vi "GUI process burst data.vi"(9 "Analysis.algo":string, 10 "TXRX data":T1, 11 "WaveformGraph in":refnum<vi>) -> (2 "Result param":string[][](array[string]), 3 "Result plot":cluster{"x0":dbl, "dx":dbl, "y":dbl[]}[](array[cluster]))   [LabVIEW 2019, in "GUI.lvlib"]
uses:
  GUI.lvlib
  SubVIs/mmWave data_class/mmWave data.lvclass
  <vilib>/Analysis/4window.llb/windowTd.ctl
  <vilib>/Analysis/coordinate.llb/Angle Units.ctl
  <vilib>/Analysis/2dsp.llb/1D Convolution (CDB).vi
  <vilib>/Analysis/coordinate.llb/Wrap Angle (array).vi
  <vilib>/measure/maspectr.llb/FFT Spectrum (Mag-Phase) for 1 Chan (CDB).vi
  <vilib>/Analysis/NI_AALPro.lvlib
  <vilib>/Analysis/NI_AAL_Angle.lvlib
  <vilib>/measure/NI_MAPro.lvlib
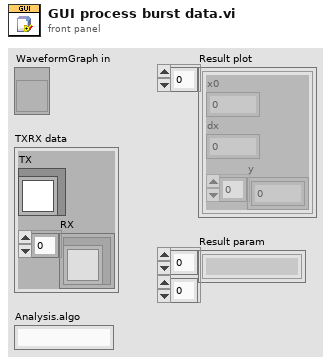
[diagram p1: front panel]
types:
  T1 = cluster{"TX":refnum<class "mmWave data.lvclass">, "RX":refnum<class "mmWave data.lvclass">[]}
  T2 = cluster{"dB On (F)":bool, "unwrap phase (F)":bool, "convert to degree (F)":bool}
  T3 = typedef "NI_AALPro.lvlib/windowTd.ctl" = u32
  T4 = typedef "NI_AAL_Angle.lvlib/Angle Units.ctl" = i32
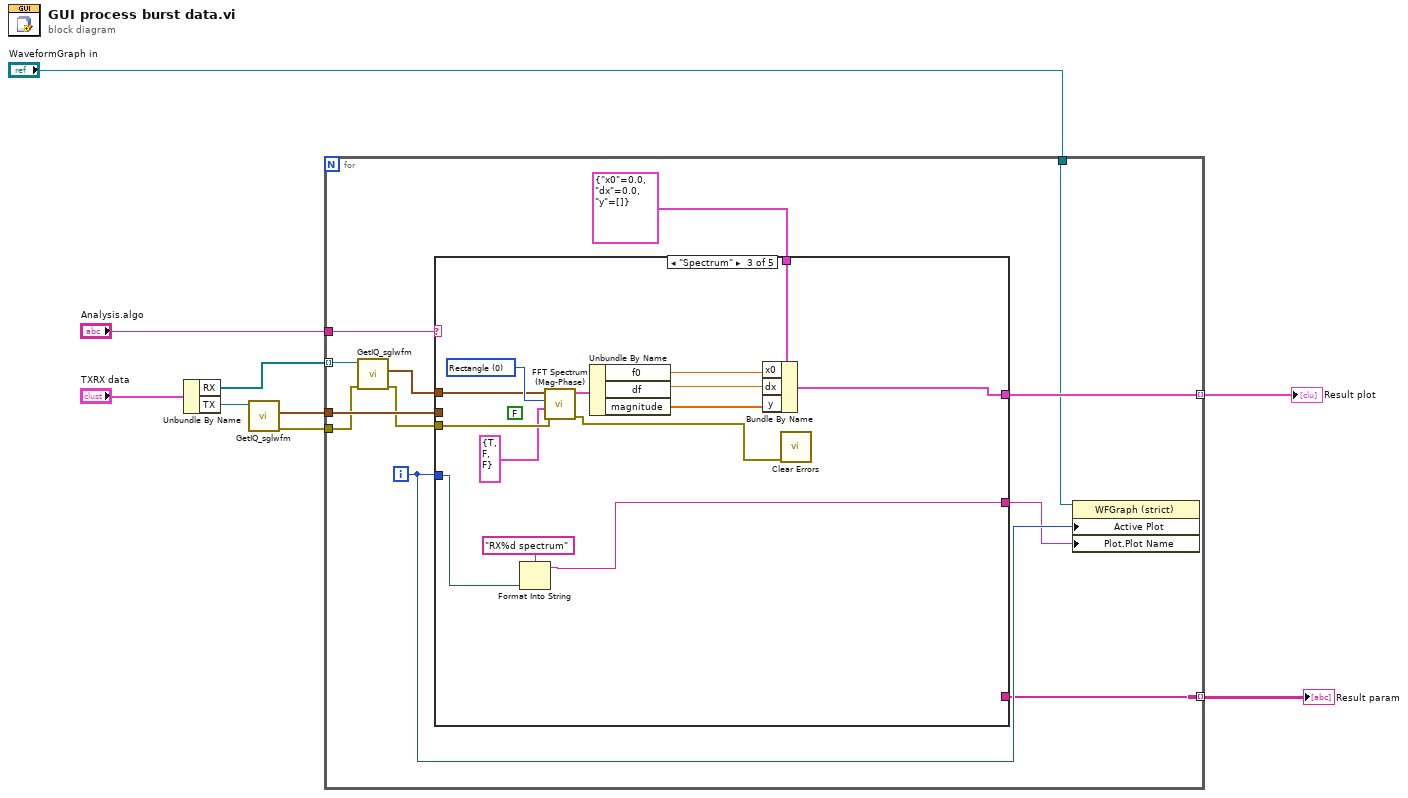
[diagram p0: block diagram]
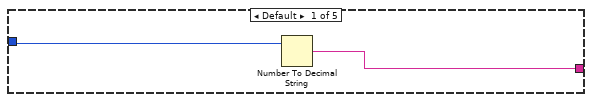
[diagram p2: hidden frame]
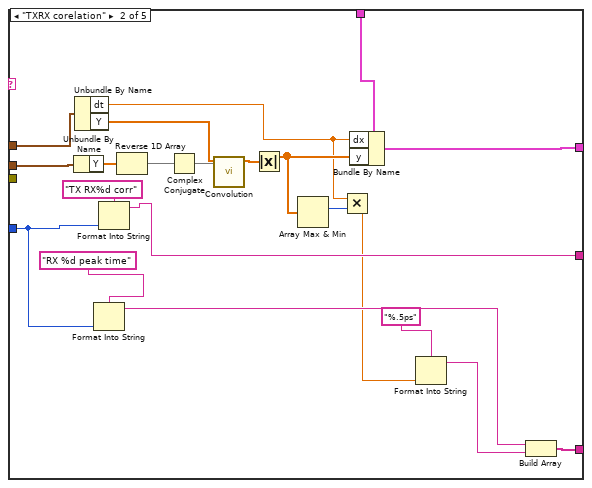
[diagram p3: hidden frame]
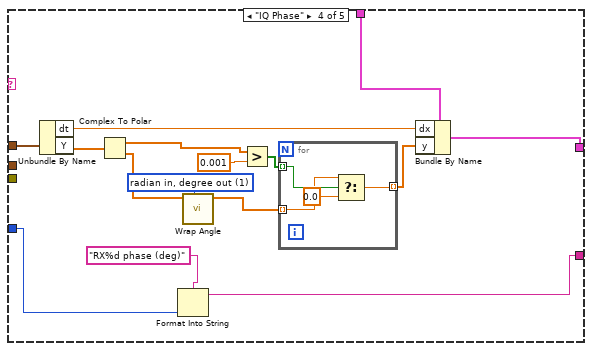
[diagram p4: hidden frame]
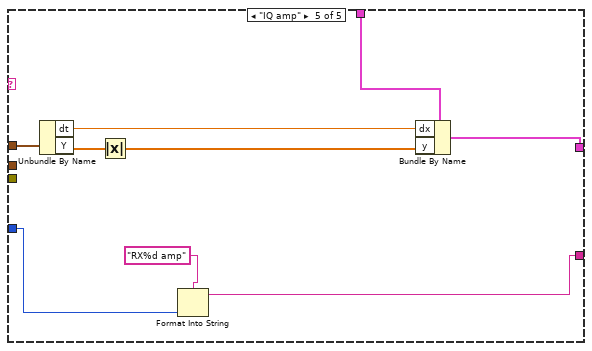
[diagram p5: hidden frame]
diagram:
  n1 = Unbundle By Name("TXRX data") -> ("RX"=w5:refnum<class "mmWave data.lvclass">[], "TX"=w4:refnum<class "mmWave data.lvclass">)
  n2 = call-dynamic "GetIQ_sglwfm.vi"("reference in"=w4) -> ("error out"=w1:errorcluster, "IQ"=w7:waveform(csg))  [unwired: 8 in, 1 out]
  n3 = for {
    tunnel: w5 -> [w21] mode=indexing
    tunnel: "Analysis.algo" -> [w20]
    tunnel: w7 -> [w19]
    tunnel: [w16] -> w8 mode=indexing
    tunnel: [w13] -> w9 mode=indexing
    tunnel: "WaveformGraph in" -> [w12]
    tunnel: w1 -> [w11]
    i -> [w17]
    n4 = call-dynamic "GetIQ_sglwfm.vi"("error in (no error)"=w11, "reference in"=w21) -> ("error out"=w10:errorcluster, "IQ"=w18:waveform(csg))  [unwired: 7 in, 1 out]
    n5 = case shown="\"Spectrum\"" w20 {
      tunnel: w19 -> [_ w41 _ _ _]
      tunnel: w18 -> [_ w38 w48 w73 w86]
      tunnel: w17 -> [w23 w29 w58 w69 w82]
      tunnel: [_ w36 w52 w70 w83] -> w16
      tunnel: cluster{"x0":dbl, "dx":dbl, "y":dbl[]} {"x0"=0.0, "dx"=0.0, "y"=[]} ("Power Spectrum / PSD") -> [_ w35 w54 w71 w84]
      tunnel: [w22 w31 w49 w67 w80] -> w14
      tunnel: [_ w30 _ _ _] -> w13
      tunnel: w10 -> [_ _ w46 _ _]
      frame Default {
        n6 = Number To Decimal String(number=w23) -> (decimal integer string=w22:string)  [unwired: 1 in]
      }
      frame "TXRX corelation" {
        n7 = Unbundle By Name(w41) -> ("Y"=w40:csg[])
        n8 = Unbundle By Name(w38) -> ("dt"=w32:dbl, "Y"=w39:csg[])
        n9 = Format Into String(format string="RX %d peak time", w29) -> (resulting string=w27:string)  [unwired: 2 in, 1 out]
        n10 = Format Into String(format string="TX RX%d corr", w29) -> (resulting string=w31:string)  [unwired: 2 in, 1 out]
        n11 = Reverse 1D Array(array=w40) -> (reversed array=w43:csg[])
        n12 = Complex Conjugate(1:w43) -> (0:w42:csg[])
        n13 = call-poly <vilib>:"Convolution.vi"("Y"=w42, "X"=w39) -> ("X * Y"=w44:cdb[])  [unwired: 8 in, 1 out]
        n14 = Absolute Value(x=w44) -> (abs(x)=w34:dbl[])
        n15 = Array Max & Min(array=w34) -> (max index (indices)=w33:i32)  [unwired: 3 out]
        n16 = Multiply(x=w32, y=w33) -> (x*y=w25:dbl)
        n17 = Bundle By Name(cluster=w35, "dx"=w32, "y"=w34) -> (w36:cluster{"x0":dbl, "dx":dbl, "y":dbl[]})
        n18 = Format Into String(format string="%.5ps", w25) -> (resulting string=w24:string)  [unwired: 2 in, 1 out]
        n19 = Build Array(w27, w24) -> (w30:string[])
      }
      frame "Spectrum" {
        (unwired) FALSE ("dB On (F)")
        w56 = T3 0 items=["Rectangle"=0, "Hanning"=1, "Hamming"=2, "Blackman-Harris"=3, "Exact Blackman"=4, "Blackman"=5, "Flat Top"=6, "4 Term B-Harris "=7, "7 Term B-Harris"=8, "Low Sidelobe"=9, "Blackman Nuttall"=11, "Triangle"=30, "Bartlett-Hanning"=31, "Bohman"=32, "Parzen"=33, "Welch"=34, "Kaiser"=60, "Dolph-Chebyshev"=61, "Gaussian"=62] ("window")
        n20 = Format Into String(format string="RX%d spectrum", w58) -> (resulting string=w49:string)  [unwired: 2 in, 1 out]
        n21 = call-poly <vilib>:"FFT Spectrum (Mag-Phase).vi"("error in (no error)"=w46, "view"=T2 {"dB On (F)"=TRUE, "unwrap phase (F)"=FALSE, "convert to degree (F)"=FALSE}, "window"=w56, "time signal"=w48) -> ("error out"=w47:errorcluster, "magnitude"=w55:cluster{"f0":dbl, "df":dbl, "magnitude":dbl[]})  [unwired: 3 in, 3 out]
        n22 = Unbundle By Name(w55) -> ("f0"=w53:dbl, "df"=w51:dbl, "magnitude"=w50:dbl[])
        n23 = Bundle By Name(cluster=w54, "x0"=w53, "dx"=w51, "y"=w50) -> (w52:cluster{"x0":dbl, "dx":dbl, "y":dbl[]})
        n24 = call <vilib>:"Clear Errors.vi"("error in (no error)"=w47) -> ()  [unwired: 5 in, 2 out]
      }
      frame "IQ Phase" {
        w59 = T4 1 items=["radian in, radian out", "radian in, degree out", "degree in, degree out", "degree in, radian out"] ("angle units")
        n25 = Unbundle By Name(w73) -> ("dt"=w65:dbl, "Y"=w72:csg[])
        n26 = Complex To Polar(r * e^(i*theta)=w72) -> (r=w64:sgl[], theta=w61:sgl[])
        n27 = Format Into String(format string="RX%d phase (deg)", w69) -> (resulting string=w67:string)  [unwired: 2 in, 1 out]
        n28 = call-poly <vilib>:"Wrap Angle.vi"("angle units"=w59, "Angle In"=w61) -> ("Angle Out"=w60:dbl[])  [unwired: 8 in, 1 out]
        n29 = Greater?(x=w64, y=0.001) -> (0:w63:bool[])
        n30 = for {
          tunnel: w63 -> [w77] mode=indexing
          tunnel: w60 -> [w76] mode=indexing
          tunnel: [w74] -> w62 mode=indexing
          n31 = Select(t=w76, s=w77, f=sgl 0.0) -> (s? t:f=w74:dbl)
        }
        n32 = Bundle By Name(cluster=w71, "dx"=w65, "y"=w62) -> (w70:cluster{"x0":dbl, "dx":dbl, "y":dbl[]})
      }
      frame "IQ amp" {
        n33 = Unbundle By Name(w86) -> ("dt"=w79:dbl, "Y"=w85:csg[])
        n34 = Absolute Value(x=w85) -> (abs(x)=w78:sgl[])
        n35 = Format Into String(format string="RX%d amp", w82) -> (resulting string=w80:string)  [unwired: 2 in, 1 out]
        n36 = Bundle By Name(cluster=w84, "dx"=w79, "y"=w78) -> (w83:cluster{"x0":dbl, "dx":dbl, "y":dbl[]})
      }
    }
    n37 = property on="Property Node" class="WFGraph (strict)"(reference=w12, "Active Plot"=w17, "Plot.Plot Name"=w14) -> ()  [unwired: 1 in, 2 out]
  }
  "Result param" <- w9
  "Result plot" <- w8
